vi "Acc processing.vi"(10 "Lower Cut-Off":dbl=5000.0 caption="하위 컷오프", 11 "Raw_acc":waveform(dbl)(graph)={"t0"=timestamp(0 s since 1904-01-01), "dt"=1e-05, "Y"=array[2000 elements]}) -> (2 "Acc_time":dbl caption="Acc time" format="%#.1p", 3 "Acc_peak":dbl=1.6258445790000002 caption="Acc peak")   [LabVIEW 2016]
uses:
  <vilib>/measure/mascope.llb/Transition Measurements 1 chan.vi
  <vilib>/Waveform/WDTOps.llb/WDT Get Waveform Subset DBL.vi
  <vilib>/measure/NI_MAPro.lvlib
panel:
  out "Y max":dbl caption="Y 최대" format="%0.2f"
  out "max time":timestamp caption="최대 시간"
  out "start time":dbl
  out "speed m/s":dbl
  in  "x":dbl
  out "웨이브폼 그래프":waveform(dbl)(graph)
  out "err out":errorcluster
  in  "error in (no error)":errorcluster caption="err in"
  out "acc wf":waveform(dbl)(graph)
  out "Filtered_acc":dynamicdata(graph)=[{"t0"=timestamp(0 s since 1904-01-01), "dt"=1e-05, "Y"=array[2000 elements], "attributes"=variant("NI_ChannelName"=variant(string "필터된"))}]
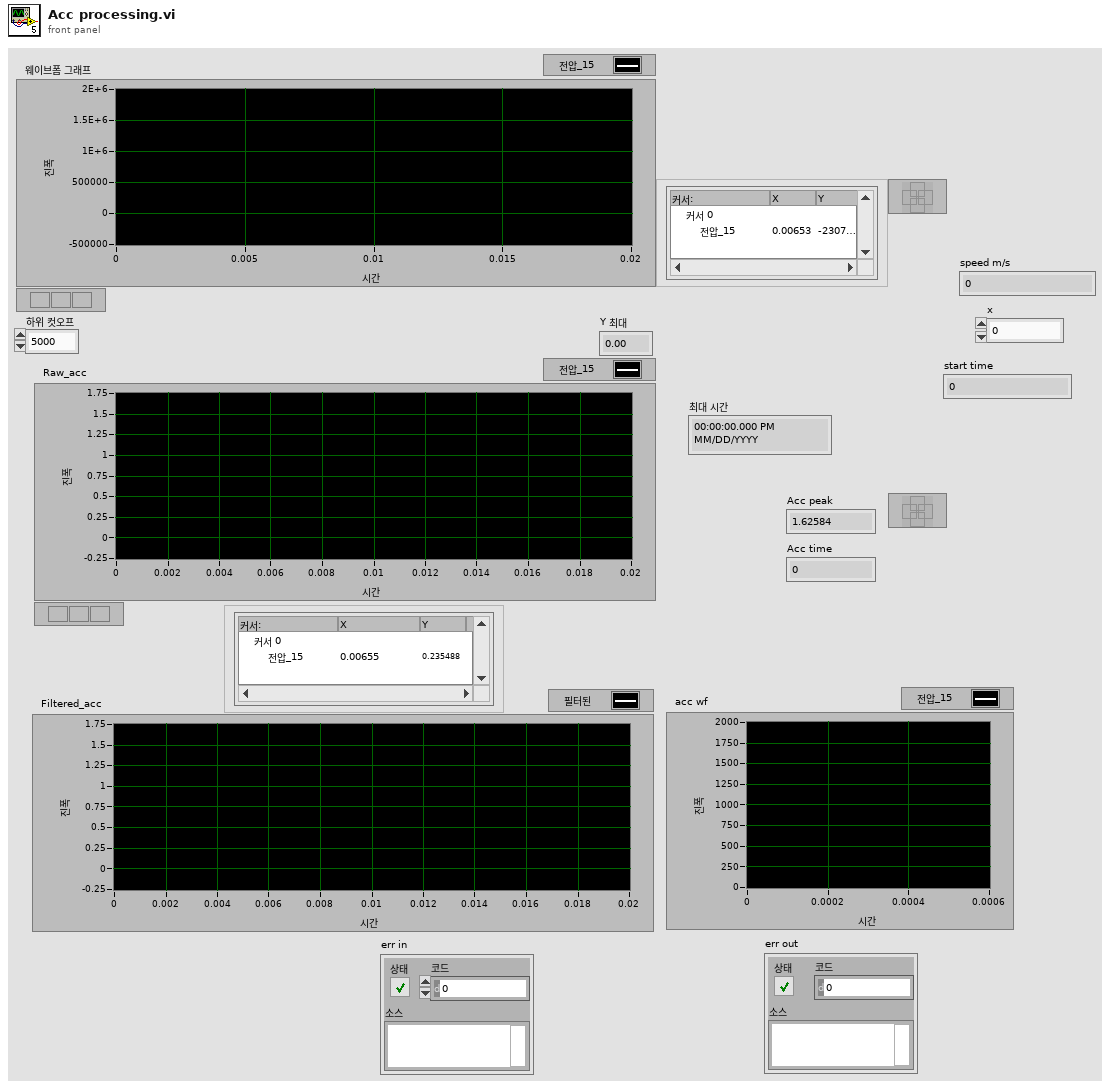
[diagram p1: front panel]
types:
  T1 = cluster{"high ref level":dbl, "mid ref level":dbl, "low ref level":dbl, "ref units":u16}
  T2 = cluster{"start time":dbl, "end time":dbl, "ref levels":cluster{"high ref level":dbl, "mid ref level":dbl, "low ref level":dbl, "ref units":u16}}
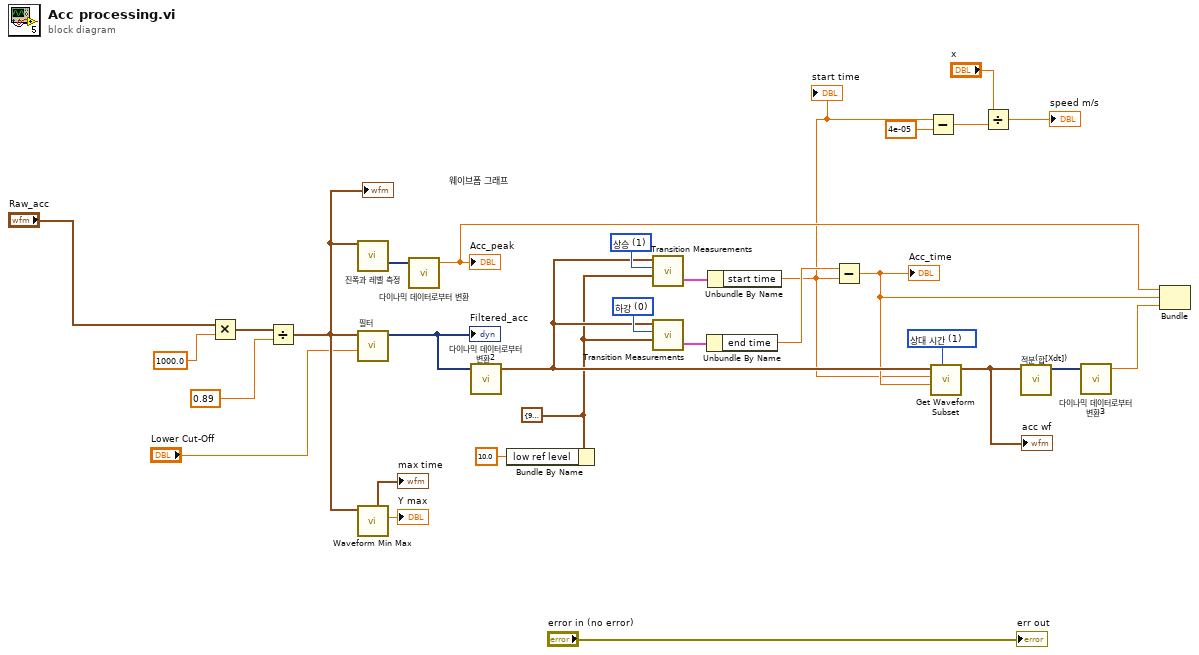
[diagram p0: block diagram]
diagram:
  w15 = T1 {"high ref level"=90.0, "mid ref level"=50.0, "low ref level"=10.0, "ref units"=1} ("reference levels")
  w22 = u16 1 items=["샘플 ", "상대 시간"] ("start/duration format")
  w28 = u16 0 items=["하강", "상승"] ("polarity (rising)")
  w29 = u16 1 items=["하강", "상승"] ("polarity (rising)")
  n1 = Multiply(x="Raw_acc", y=1000.0) -> (x*y=w13:waveform(dbl))
  n2 = Divide(x=w13, y=0.89) -> (x/y=w4:waveform(dbl))
  "웨이브폼 그래프" <- w4
  n3 = call "진폭과 레벨 측정"("Signals"=w4) -> ("Positive Peak"=w30:dynamicdata)  [unwired: 13 in, 1 out]
  n4 = call "필터"("Lower Cut-Off"="Lower Cut-Off", "Signal"=w4) -> ("Filtered Signal"=w24:dynamicdata)  [unwired: 8 in, 1 out]
  "Filtered_acc" <- w24
  n5 = call <vilib>:"Waveform Min Max.vi"("waveform in"=w4) -> ("Y max"=→"Y max":dbl, "max time"=→"max time":timestamp)  [unwired: 5 in, 4 out]
  n6 = call "다이나믹 데이터로부터 변환"("Dynamic Data Type"=w30) -> ("Scalar"=w19:dbl)  [unwired: 3 in]
  "Acc_peak" <- w19
  n7 = call "다이나믹 데이터로부터 변환2"("Dynamic Data Type"=w24) -> ("Waveform"=w23:waveform(dbl))  [unwired: 3 in]
  n8 = Bundle By Name(cluster=w15, "low ref level"=10.0) -> ()  [unwired: 1 out]
  n9 = call-poly <vilib>:"Transition Measurements.vi"("reference levels"=w15, "polarity (rising)"=w29, "signal in"=w23) -> ("measurement info"=w27:T2)  [unwired: 3 in, 5 out]
  n10 = call-poly <vilib>:"Transition Measurements.vi"("reference levels"=w15, "polarity (rising)"=w28, "signal in"=w23) -> ("measurement info"=w26:T2)  [unwired: 3 in, 5 out]
  n11 = Unbundle By Name(w26) -> ("end time"=w25:dbl)
  n12 = Unbundle By Name(w27) -> ("start time"=w9:dbl)
  "start time" <- w9
  n13 = Subtract(x=w25, y=w9) -> (x-y=w18:dbl)
  "Acc_time" <- w18
  n14 = Subtract(x=w9, y=4e-05) -> (x-y=w7:dbl)
  n15 = call-poly <vilib>:"Get Waveform Subset.vi"("start/duration format"=w22, "duration"=w18, "start samples/time"=w9, "waveform in"=w23) -> ("waveform out"=w21:waveform(dbl))  [unwired: 2 in, 3 out]
  "acc wf" <- w21
  n16 = Divide(x="x", y=w7) -> (x/y=→"speed m/s":dbl)
  n17 = call "적분(합[Xdt])"("Signals"=w21) -> ("Result"=w20:dynamicdata)  [unwired: 5 in, 1 out]
  n18 = call "다이나믹 데이터로부터 변환3"("Dynamic Data Type"=w20) -> ("Scalar"=w16:dbl)  [unwired: 3 in]
  n19 = Bundle("Scalar"=w19, w18, "Scalar"=w16) -> ()  [unwired: 1 in, 1 out]
  "err out" <- "error in (no error)"
